vi "trackFaces.vi"(4 "WiFi Info":T2={"WiFi"={"SSID"="", "Key"=""}, "SystemLink"={"APIKey"="", "Tag"="", "Type"="STRING"}}, 5 "ROI":T1, 6 "Output":enum16{"None", "UART", "SPI", "I2C", "WiFi"}(ring), 8 "error in (no error)":errorcluster, 10 "Value":enum16{"# faces", "All data"}(ring), 11 "VISA Refnum in":refnum<visa-resource-name>) -> (0 "error out":errorcluster, 2 "Python Code":string, 3 "VISA Refnum out":refnum<visa-resource-name>)   [LabVIEW 2017]
uses:
  <userlib>/LabVIEWOpenMV/_subs/CameraSetup.ctl
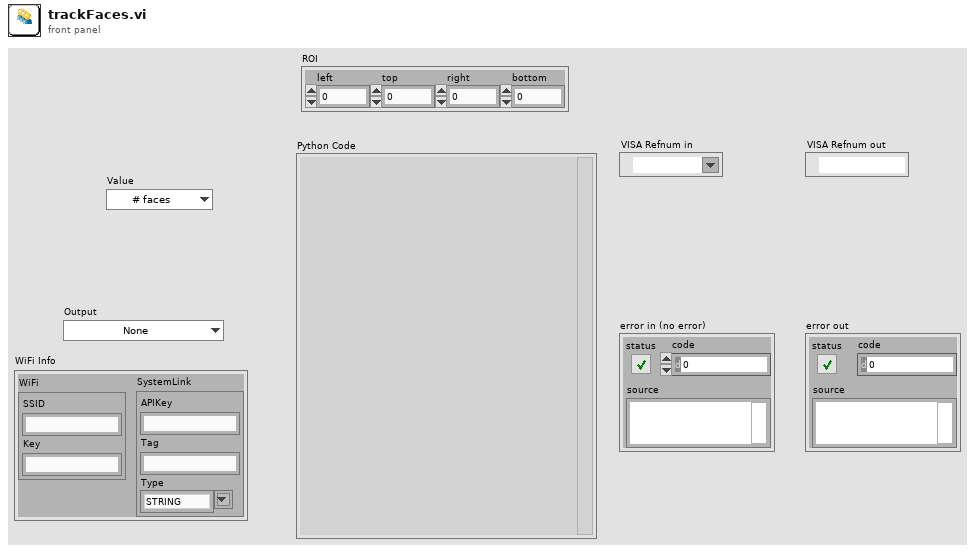
[diagram p1: front panel]
types:
  T1 = cluster{"left":i32, "top":i32, "right":i32, "bottom":i32}
  T2 = cluster{"WiFi":cluster{"SSID":string, "Key":string}, "SystemLink":cluster{"APIKey":string, "Tag":string, "Type":string}}
  T3 = typedef "CameraSetup.ctl" = cluster{"Format":enum16{"GRAYSCALE", "RGB565", "BAYER"}, "size":enum16{"QQQQVGA (40x30)", "QQQVGA (80x60)", "QQVGA (160x120)", "QVGA (320x240)", "VGA (640x480)", "LCD (128x160)", "B64x32 (64x32)", "B64x64", "B128x64", "B128x128"}, "Skip frames (ms)":u16, "autoGain":bool, "autoWhitebal":bool}
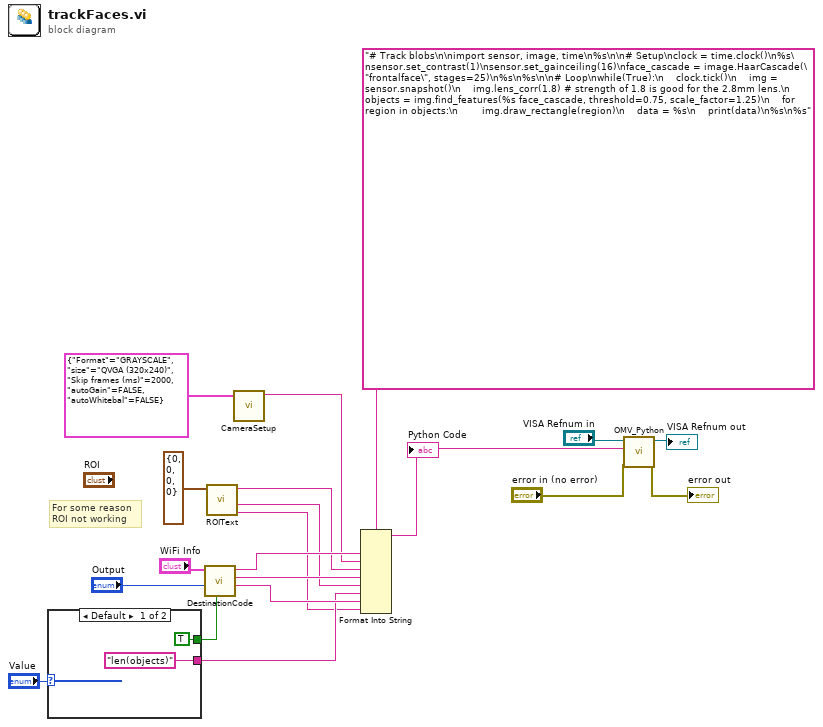
[diagram p0: block diagram]
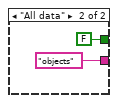
[diagram p2: hidden frame]
diagram:
  # "For some reason\nROI not working"
  n1 = case shown="Default" "Value" {
    tunnel: ["len(objects)" "objects"] -> w6
    tunnel: [TRUE FALSE] -> w1
    frame Default {
    }
    frame "All data" {
    }
  }
  n2 = call <userlib>:"DestinationCode.vi"("Single number?"=w1, "Destination"="Output", "WiFi Info"="WiFi Info") -> ("Repeated call"=w17:string, "Setup"=w18:string, "Headers"=w15:string)  [unwired: 6 in]
  n3 = call <userlib>:"ROIText.vi"("ROI"=T1 {"left"=0, "top"=0, "right"=0, "bottom"=0}) -> ("draw"=w3:string, "with comma"=w2:string, "r"=w4:string)  [unwired: 7 in, 1 out]
  n4 = call <userlib>:"CameraSetup.vi"("Camera Setup"=T3 {"Format"=enum."GRAYSCALE", "size"=enum."QVGA (320x240)", "Skip frames (ms)"=2000, "autoGain"=FALSE, "autoWhitebal"=FALSE}) -> ("String"=w14:string)  [unwired: 10 in]
  n5 = Format Into String(format string="# Track blobs\n\nimport sensor, image, time\n%s\n\n# Setup\nclock = time.clock()\n%s\nsensor.set_contrast(1)\nsensor.set_gainceiling(16)\nface_cascade = image.HaarCascade(\"frontalface\", stages=25)\n%s\n%s\n\n# Loop\nwhile(True):\n    clock.tick()\n    img = sensor.snapshot()\n    img.lens_corr(1.8) # strength of 1.8 is good for the 2.8mm lens.\n    objects = img.find_features(%s face_cascade, threshold=0.75, scale_factor=1.25)\n    for region in objects:\n        img.draw_rectangle(region)\n    data = %s\n    print(data)\n%s\n%s" ("startCode"), w15, w14, w4, w18, w2, w6, w17, w3) -> (resulting string=w8:string)  [unwired: 2 in, 1 out]
  "Python Code" <- w8
  n6 = call <userlib>:"OMV_Python.vi"("error in (no error)"="error in (no error)", "Script"=w8, "VISA Refnum in"="VISA Refnum in") -> ("error out"=→"error out":errorcluster, "VISA Refnum out"=→"VISA Refnum out":refnum<visa-resource-name>)  [unwired: 7 in]
